vi "PGPASS.Format Connection String with Password.vi"(8 "error in":errorcluster, 11 "Connection Information":T1) -> (0 "error out":errorcluster, 3 "connection string":string)   [LabVIEW 2019, in "PGPASS.lvlib"]
uses:
  PGPASS.Connection Information.ctl
  PGPASS.lvlib
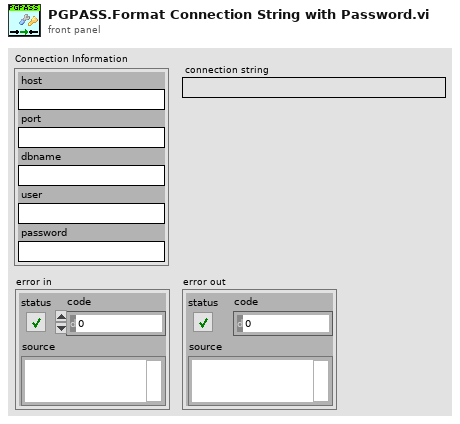
[diagram p1: front panel]
types:
  T1 = typedef "PGPASS.lvlib/PGPASS.Connection Information.ctl" = cluster{"host":string, "port":string, "dbname":string, "user":string, "password":string}
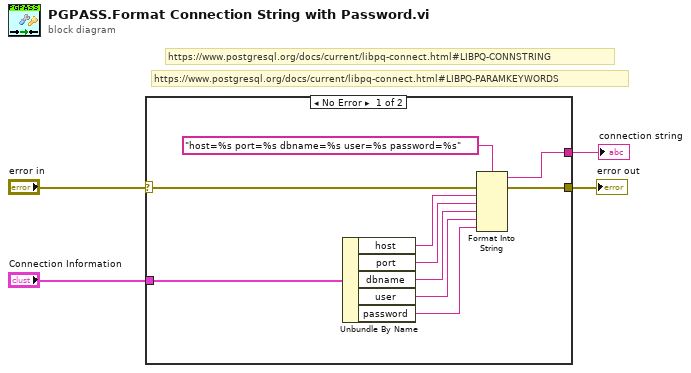
[diagram p0: block diagram]
diagram:
  # "https://www.postgresql.org/docs/current/libpq-connect.html#LIBPQ-PARAMKEYWORDS"
  # "https://www.postgresql.org/docs/current/libpq-connect.html#LIBPQ-CONNSTRING"
  n1 = case shown="No Error" "error in" {
    selector: "error in" -> [w6 w15]
    tunnel: "Connection Information" -> [w13 _]
    tunnel: [w8 _] -> w3
    tunnel: [w7 w15] -> w2
    frame No Error {
      n2 = Unbundle By Name(w13) -> ("host"=w12:string, "port"=w11:string, "dbname"=w10:string, "user"=w9:string, "password"=w5:string)
      n3 = Format Into String(format string="host=%s port=%s dbname=%s user=%s password=%s", error in=w6, w12, w11, w10, w9, w5) -> (resulting string=w8:string, error out=w7:errorcluster)  [unwired: 1 in]
    }
    frame Error {
    }
  }
  "connection string" <- w3
  "error out" <- w2
